vi "Get Min Attenuation.vi"(8 "error in (no error)":errorcluster, 11 "Device ID in":i32) -> (0 "error out":errorcluster, 2 "Min Attenuation (dB)":dbl, 3 "Device ID out":i32)   [LabVIEW 2013, in "Vaunix LDA.lvlib"]
doc: "VNX_ATTEN_API int fnLDA_GetMinAttenuation(DEVID deviceID)\n\nThis function returns the minimum attenuation value that the device can provide. For the LDA-102 and LDA-602 programmable attenuators this value is 0 db. Since future products may have different capabilities your software should use this function to obtain the minimum attenuation possible.\n\nNote: The VI converts from what the function returns into Engineering units of dB."
uses:
  Attenuator_Vaunix-LDA_LabView_32Bit_Driver/Vaunix LDA/Vaunix LDA.lvlib
  Attenuator_Vaunix-LDA_LabView_32Bit_Driver/Vaunix LDA/VNX_atten.dll
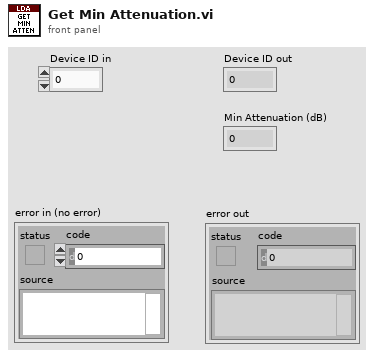
[diagram p1: front panel]
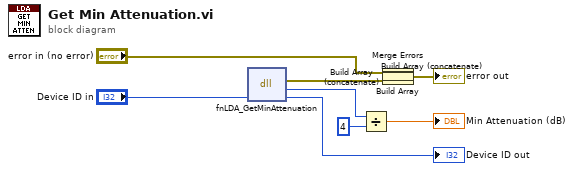
[diagram p0: block diagram]
diagram:
  n1 = dll-call lib="C:/Users/manip.batm/Desktop/FPGA_Batch_1_7_3/Attenuator_Vaunix-LDA_LabView_32Bit_Driver/Vaunix LDA/VNX_atten.dll" fn="fnLDA_GetMinAttenuation"("deviceID"="Device ID in") -> (error out=w9:errorcluster, "attenuation"=w8:i32, "deviceID"=→"Device ID out":i32)  [unwired: 3 in, 1 out]
  n2 = Divide(x=w8, y=4) -> (x/y=→"Min Attenuation (dB)":dbl)
  n3 = Build Array("error in (no error)", w9) -> (w3:errorcluster[])
  n4 = Build Array (concatenate)(w3) -> (w2:errorcluster[])
  n5 = Build Array (concatenate)(w2) -> (w1:errorcluster[])
  n6 = Merge Errors(w1) -> (→"error out":errorcluster)
